vi "XIPIN_3GPP_Mixed_Mode_Turbo_Decoder_2_0.vi"   [LabVIEW 2017]
doc: "The Turbo Decoder IP core from Xilinx is a high-performance, compact Turbo Decoder which meets both the 3GPP LTE and UMTS specifications. The core is delivered through the Vivado IP Catalog and integrates seamlessly with the Xilinx design flow.\n------------------------------------\n<b>Need License</b> : Yes\n<b>Interface</b> : AXI4-Stream"
uses:
  <vilib>/rvi/XilinxIP/XIPIN_XNode/niFpgaXIPIN.xnode
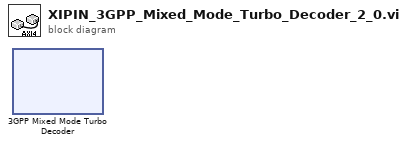
[diagram p0: block diagram]
diagram:
  n1 = xnode ("3GPP Mixed Mode Turbo Decoder")() -> ()
